vi "Cheby Tn(x).vi"(1 "n":u32, 2 "x":dbl format="%.2f") -> (0 "T(n,x)":dbl format="%.2f")   [LabVIEW 2025]
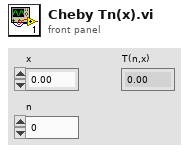
[diagram p1: front panel]
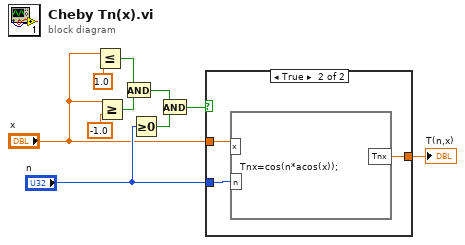
[diagram p0: block diagram]
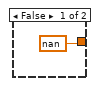
[diagram p2: hidden frame]
diagram:
  n1 = Less Or Equal?(x="x", y=1.0) -> (x <= y?=w2:bool)
  n2 = Greater Or Equal?(x="x", y=-1.0) -> (x >= y?=w3:bool)
  n3 = And(x=w2, y=w3) -> (x .and. y?=w1:bool)
  n4 = Greater Or Equal To 0?(x="n") -> (x >= 0?=w9:bool)
  n5 = And(x=w1, y=w9) -> (x .and. y?=w7:bool)
  n6 = case shown="True" w7 {
    tunnel: "x" -> [_ w14]
    tunnel: "n" -> [_ w13]
    tunnel: [nan w12] -> w10
    frame False {
    }
    frame True {
      n7 = formula code="Tnx=cos(n*acos(x));"("x"=w14, "n"=w13) -> ("Tnx"=w12:dbl)
    }
  }
  "T(n,x)" <- w10
